vi "Select Display Screen.vi"(8 "error in (no error)":errorcluster, 10 "Screen Home":u16(ring) items=["Home Screen", "Home Large Reading", "Reading Sheet", "Graph Screen", "Histogram", "Functions Swipe", "Graph Swipe", "Secondary Swipe", "Settings Swipe", "Statistics Swipe", "User Swipe"], 11 "VISA resource name":refnum<visa-resource-name>) -> (0 "error out":errorcluster, 3 "VISA resource name out":refnum<visa-resource-name>)   [LabVIEW 2018, in "Keithley DMM7512.lvlib"]
doc: "Enables or disables the display on the front of the instrument. Disabling the display can result in faster measurements."
uses:
  <instrlib>/Keithley DMM7512/Keithley DMM7512.lvlib
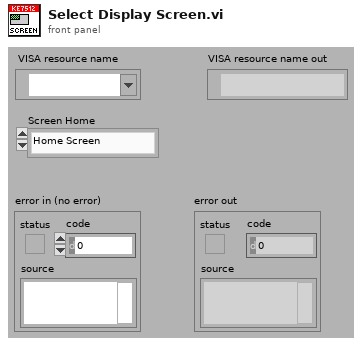
[diagram p1: front panel]
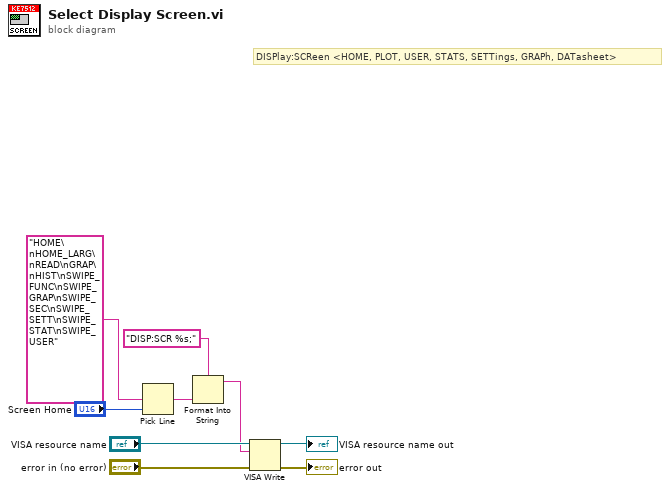
[diagram p0: block diagram]
diagram:
  # "DISPlay:SCReen <HOME, PLOT, USER, STATS, SETTings, GRAPh, DATasheet>"
  n1 = Pick Line(multi-line string="HOME\nHOME_LARG\nREAD\nGRAP\nHIST\nSWIPE_FUNC\nSWIPE_GRAP\nSWIPE_SEC\nSWIPE_SETT\nSWIPE_STAT\nSWIPE_USER", line index="Screen Home") -> (output string=w1:string)  [unwired: 1 in]
  n2 = Format Into String(format string="DISP:SCR %s;", w1) -> (resulting string=w4:string)  [unwired: 2 in, 1 out]
  n3 = VISA Write(VISA resource name="VISA resource name", write buffer=w4, error in (no error)="error in (no error)") -> (VISA resource name out=→"VISA resource name out":refnum<visa-resource-name>, error out=→"error out":errorcluster)  [unwired: 1 out]
